vi "writeNewScripts.vi"(8 "error in (no error)":errorcluster, 10 "delayAll":bool, 11 "ScanCreator in":refnum<class "ScanCreator.lvclass">) -> (0 "error out":errorcluster, 1 "Values":string[](array[string]), 2 "scriptListArray":refnum<class "ScriptEventList.lvclass">[](array[class]), 3 "ScanCreator out":refnum<class "ScanCreator.lvclass">, 4 "scanType":string)   [LabVIEW 2009, in "Views.lvlib" / "ScriptEditor.lvlib" / "ScanCreator.lvclass"]
uses:
  ScanCreator.lvclass
  Tools/Scripting/ScriptingEvent/ScriptEventList/ScriptEventList.lvclass
  ScanCreator.lvclass/ScanCreator.ctl
  Tools/Scripting/ScriptingEvent/ScriptEvent.lvclass
  Tools/Scripting/ScriptingEvent/ScriptEvents/Ramp/RampEvent/RampEvent.lvclass
  Tools/Scripting/ScriptingEvent/ScriptEvents/Rf Event/rf.lvclass
  Tools/DatabaseHelpers/Database Objects/Channel/Channel.lvclass
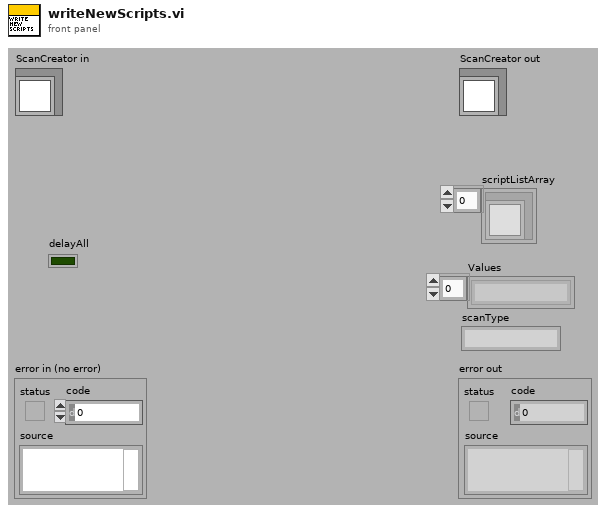
[diagram p1: front panel]
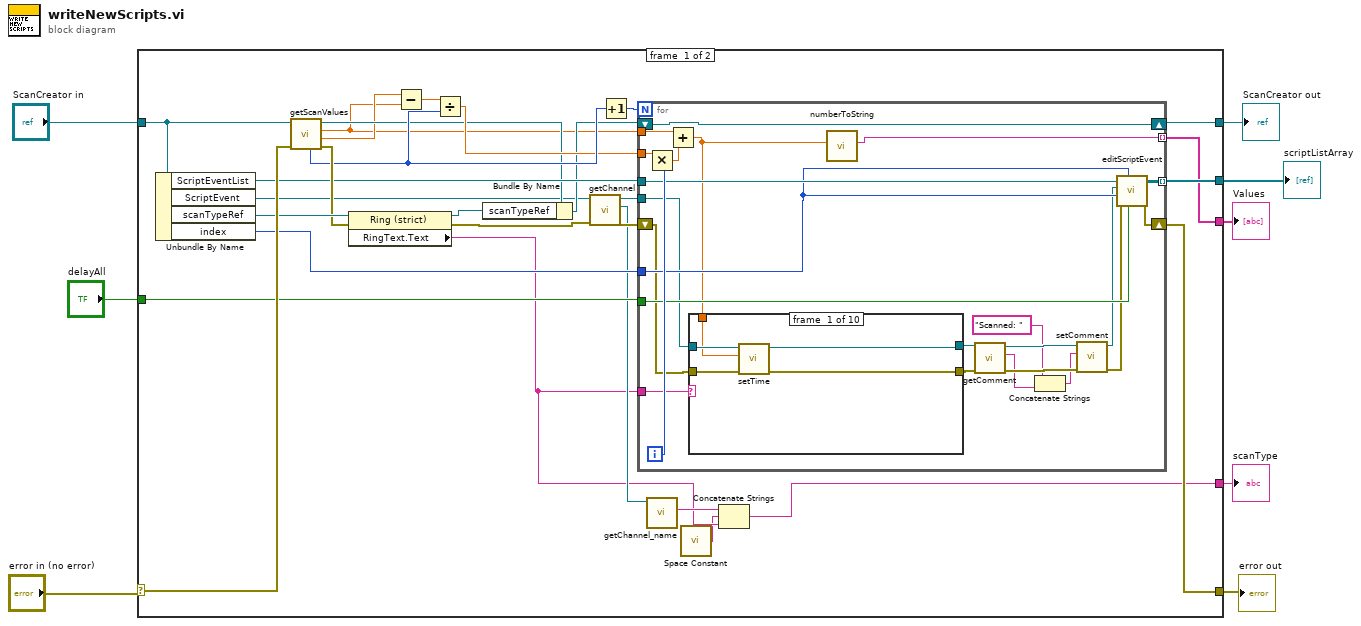
[diagram p0: block diagram]
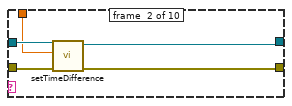
[diagram p2: hidden frame]
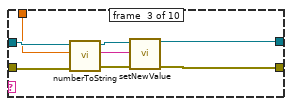
[diagram p3: hidden frame]
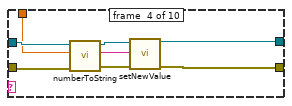
[diagram p4: hidden frame]
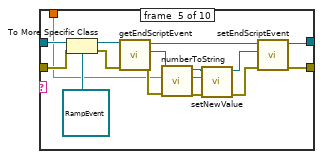
[diagram p5: hidden frame]
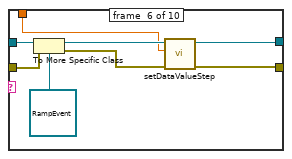
[diagram p6: hidden frame]
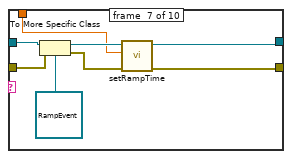
[diagram p7: hidden frame]
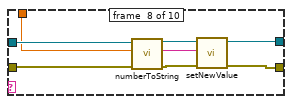
[diagram p8: hidden frame]
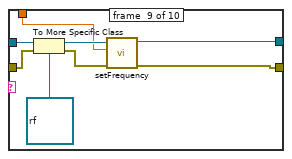
[diagram p9: hidden frame]
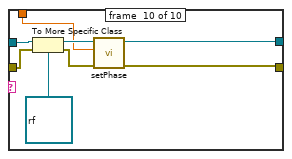
[diagram p10: hidden frame]
diagram:
  n1 = case shown="No Error" "error in (no error)" {
    selector: "error in (no error)" -> [w36 w145]
    tunnel: [w22 w145] -> w7
    tunnel: [w26 w144] -> w5
    tunnel: "ScanCreator in" -> [w37 w144]
    tunnel: "delayAll" -> [w28 _]
    tunnel: [w27 _] -> w3
    tunnel: [w20 _] -> w2
    tunnel: [w10 _] -> w1
    frame #0 {
      n2 = Unbundle By Name(w37) -> ("ScriptEventList"=w33:refnum<class "ScriptEventList.lvclass">, "ScriptEvent"=w15:refnum<class "ScriptEvent.lvclass">, "scanTypeRef"=w35:refnum<vi>, "index"=w29:i16)
      n3 = call "getScanValues.vi"("error in (no error)"=w36, "ScanCreator in"=w37) -> ("error out"=w34:errorcluster, "stop"=w19:dbl, "start"=w18:dbl, "ScanCreator out"=w25:refnum<class "ScanCreator.lvclass">, "step"=w31:i16)  [unwired: 5 in]
      n4 = property class="Ring (strict)"(reference=w35, error in=w34) -> (reference out=w23:refnum<vi>, error out=w16:errorcluster, "RingText.Text"=w11:string)
      n5 = Subtract(x=w19, y=w18) -> (x-y=w32:dbl)
      n6 = Divide(x=w32, y=w31) -> (x/y=w30:dbl)
      n7 = Bundle By Name(cluster=w25, "scanTypeRef"=w23) -> (w24:refnum<class "ScanCreator.lvclass">)
      n8 = call-dynamic "getChannel.vi"("error in (no error)"=w16, "ScriptEvent.lvclass in"=w15) -> ("error out"=w17:errorcluster, "Channel.lvclass"=w13:refnum<class "Channel.lvclass">, "ScriptEvent.lvclass out"=w14:refnum<class "ScriptEvent.lvclass">)  [unwired: 7 in]
      n9 = Increment(x=w31) -> (x+1=w21:i16)
      n10 = for {
        N: w21 -> [_]
        tunnel: w30 -> [w60]
        tunnel: w14 -> [w51]
        tunnel: w18 -> [w61]
        tunnel: w33 -> [w57]
        tunnel: w29 -> [w56]
        tunnel: w28 -> [w55]
        tunnel: [w54] -> w27 mode=indexing
        shift-right: [w53] -> w22
        shift-left: w17 -> [w50]
        shift-right: [w52] -> w26
        shift-left: w24 -> [w52]
        tunnel: w11 -> [w49]
        tunnel: [w47] -> w20 mode=indexing
        i -> [w59]
        n11 = Multiply(x=w60, y=w59) -> (x*y=w58:dbl)
        n12 = Add(x=w61, y=w58) -> (x+y=w48:dbl)
        n13 = case shown="\"Start Value\"" w49 {
          tunnel: w51 -> [w66 w71 w73 w81 w103 w110 w118 w127 w135 w142]
          tunnel: w50 -> [w63 w70 w74 w82 w101 w109 w117 w121 w134 w141]
          tunnel: [w64 w67 w78 w86 w92 w106 w112 w124 w128 w136] -> w45
          tunnel: [w65 w68 w79 w87 w90 w107 w113 w125 w129 w137] -> w46
          tunnel: w48 -> [w62 w69 w72 w80 w96 w105 w114 w120 w130 w138]
          frame #0 {
            n14 = call "setTime.vi"("error in (no error)"=w63, "time"=w62, "ScriptEvent.lvclass in"=w66) -> ("error out"=w64:errorcluster, "ScriptEvent.lvclass out"=w65:refnum<class "ScriptEvent.lvclass">)  [unwired: 7 in]
          }
          frame #1 {
            n15 = call "setTimeDifference.vi"("error in (no error)"=w70, "time difference"=w69, "ScriptEvent.lvclass in"=w71) -> ("error out"=w67:errorcluster, "ScriptEvent.lvclass out"=w68:refnum<class "ScriptEvent.lvclass">)  [unwired: 7 in]
          }
          frame #2 {
            n16 = call "numberToString.vi"("error in (no error)"=w74, "Numeric"=w72, "ScriptEvent in"=w73) -> ("error out"=w75:errorcluster, "String"=w76:string, "ScriptEvent out"=w77:refnum<class "ScriptEvent.lvclass">)  [unwired: 6 in]
            n17 = call "setNewValue.vi"("error in (no error)"=w75, "newValue"=w76, "ScriptEvent.lvclass in"=w77) -> ("error out"=w78:errorcluster, "ScriptEvent.lvclass out"=w79:refnum<class "ScriptEvent.lvclass">)  [unwired: 7 in]
          }
          frame #3 {
            n18 = call "numberToString.vi"("error in (no error)"=w82, "Numeric"=w80, "ScriptEvent in"=w81) -> ("error out"=w83:errorcluster, "String"=w84:string, "ScriptEvent out"=w85:refnum<class "ScriptEvent.lvclass">)  [unwired: 6 in]
            n19 = call "setNewValue.vi"("error in (no error)"=w83, "newValue"=w84, "ScriptEvent.lvclass in"=w85) -> ("error out"=w86:errorcluster, "ScriptEvent.lvclass out"=w87:refnum<class "ScriptEvent.lvclass">)  [unwired: 7 in]
          }
          frame #4 {
            n20 = To More Specific Class(target class=refnum<class "RampEvent.lvclass"> refnum ("Tools.lvlib:Scripting.lvlib:RampEvent.lvclass"), reference=w103, error in=w101) -> (specific class reference=w100:refnum<class "RampEvent.lvclass">, error out=w99:errorcluster)
            n21 = call "getEndScriptEvent.vi"("error in (no error)"=w99, "RampEvent.lvclass in"=w100) -> ("error out"=w97:errorcluster, "ScriptEvent.lvclass"=w98:refnum<class "ScriptEvent.lvclass">, "RampEvent.lvclass out"=w91:refnum<class "RampEvent.lvclass">)  [unwired: 7 in]
            n22 = call "numberToString.vi"("error in (no error)"=w97, "Numeric"=w96, "ScriptEvent in"=w98) -> ("error out"=w94:errorcluster, "String"=w93:string, "ScriptEvent out"=w95:refnum<class "ScriptEvent.lvclass">)  [unwired: 6 in]
            n23 = call "setNewValue.vi"("error in (no error)"=w94, "newValue"=w93, "ScriptEvent.lvclass in"=w95) -> ("error out"=w89:errorcluster, "ScriptEvent.lvclass out"=w88:refnum<class "ScriptEvent.lvclass">)  [unwired: 7 in]
            n24 = call "setEndScriptEvent.vi"("error in (no error)"=w89, "endScriptEvent.lvclass"=w88, "RampEvent.lvclass in"=w91) -> ("error out"=w92:errorcluster, "RampEvent.lvclass out"=w90:refnum<class "RampEvent.lvclass">)  [unwired: 7 in]
          }
          frame #5 {
            n25 = To More Specific Class(target class=refnum<class "RampEvent.lvclass"> refnum ("Tools.lvlib:Scripting.lvlib:RampEvent.lvclass"), reference=w110, error in=w109) -> (specific class reference=w108:refnum<class "RampEvent.lvclass">, error out=w104:errorcluster)
            n26 = call "setDataValueStep.vi"("error in (no error)"=w104, "dataValueStep"=w105, "RampEvent.lvclass in"=w108) -> ("error out"=w106:errorcluster, "RampEvent.lvclass out"=w107:refnum<class "RampEvent.lvclass">)  [unwired: 7 in]
          }
          frame #6 {
            n27 = To More Specific Class(target class=refnum<class "RampEvent.lvclass"> refnum ("Tools.lvlib:Scripting.lvlib:RampEvent.lvclass"), reference=w118, error in=w117) -> (specific class reference=w116:refnum<class "RampEvent.lvclass">, error out=w115:errorcluster)
            n28 = call "setRampTime.vi"("error in (no error)"=w115, "rampTime"=w114, "RampEvent.lvclass in"=w116) -> ("error out"=w112:errorcluster, "RampEvent.lvclass out"=w113:refnum<class "RampEvent.lvclass">)  [unwired: 7 in]
          }
          frame #7 {
            n29 = call "numberToString.vi"("error in (no error)"=w121, "Numeric"=w120, "ScriptEvent in"=w127) -> ("error out"=w123:errorcluster, "String"=w122:string, "ScriptEvent out"=w126:refnum<class "ScriptEvent.lvclass">)  [unwired: 6 in]
            n30 = call "setNewValue.vi"("error in (no error)"=w123, "newValue"=w122, "ScriptEvent.lvclass in"=w126) -> ("error out"=w124:errorcluster, "ScriptEvent.lvclass out"=w125:refnum<class "ScriptEvent.lvclass">)  [unwired: 7 in]
          }
          frame #8 {
            n31 = To More Specific Class(target class=refnum<class "rf.lvclass"> refnum ("Tools.lvlib:Scripting.lvlib:rf.lvclass"), reference=w135, error in=w134) -> (specific class reference=w132:refnum<class "rf.lvclass">, error out=w131:errorcluster)
            n32 = call "setFrequency.vi"("error in (no error)"=w131, "frequency"=w130, "rf in"=w132) -> ("error out"=w128:errorcluster, "rf out"=w129:refnum<class "rf.lvclass">)  [unwired: 7 in]
          }
          frame #9 {
            n33 = To More Specific Class(target class=refnum<class "rf.lvclass"> refnum ("Tools.lvlib:Scripting.lvlib:rf.lvclass"), reference=w142, error in=w141) -> (specific class reference=w140:refnum<class "rf.lvclass">, error out=w139:errorcluster)
            n34 = call "setPhase.vi"("error in (no error)"=w139, "phase"=w138, "rf in"=w140) -> ("error out"=w136:errorcluster, "rf out"=w137:refnum<class "rf.lvclass">)  [unwired: 7 in]
          }
        }
        n35 = call "numberToString.vi"("Numeric"=w48) -> ("String"=w47:string)  [unwired: 8 in, 2 out]
        n36 = call "getComment.vi"("error in (no error)"=w45, "ScriptEvent.lvclass in"=w46) -> ("error out"=w43:errorcluster, "comment"=w42:string, "ScriptEvent.lvclass out"=w44:refnum<class "ScriptEvent.lvclass">)  [unwired: 7 in]
        n37 = Concatenate Strings("Scanned: ", w42) -> (w40:string)
        n38 = call-dynamic "setComment.vi"("error in (no error)"=w43, "comment"=w40, "ScriptEvent.lvclass in"=w44) -> ("error out"=w38:errorcluster, "ScriptEvent.lvclass out"=w39:refnum<class "ScriptEvent.lvclass">)  [unwired: 7 in]
        n39 = call "editScriptEvent.vi"("delayAll"=w55, "selectedIndex"=w56, "error in (no error)"=w38, "index"=w56, "ScriptEvent"=w39, "ScriptEventList in"=w57) -> ("error out"=w53:errorcluster, "ScriptEventList out"=w54:refnum<class "ScriptEventList.lvclass">)  [unwired: 4 in]
      }
      n40 = call "getChannel_name.vi"("Channel.lvclass in"=w13) -> ("channel_name"=w12:string)  [unwired: 8 in, 2 out]
      n41 = call <vilib>:"Space Constant.vi"() -> ("String"=w9:string)
      n42 = Concatenate Strings(w12, w9, w11) -> (w10:string)
    }
    frame #1 {
    }
  }
  "error out" <- w7
  "ScanCreator out" <- w5
  "scriptListArray" <- w3
  "Values" <- w2
  "scanType" <- w1
